vi "Begin.vi"(8 "error in (no error)":errorcluster, 11 "DriveMotors in":refnum<class "DriveMotors.lvclass">) -> (0 "error out":errorcluster, 3 "DriveMotors out":refnum<class "DriveMotors.lvclass">)   [LabVIEW 2013, in "DriveMotors.lvclass"]
uses:
  DriveMotors.lvclass
  DriveMotors.lvclass/DriveMotors.ctl
  System/System.lvclass
  <vilib>/Rock Robotics/WPI/Counter/WPI_CounterDigitalInputToDigitalSource.vi
  <vilib>/Rock Robotics/WPI/MotorControl/WPI_MotorControlOpenCANJaguar.vi
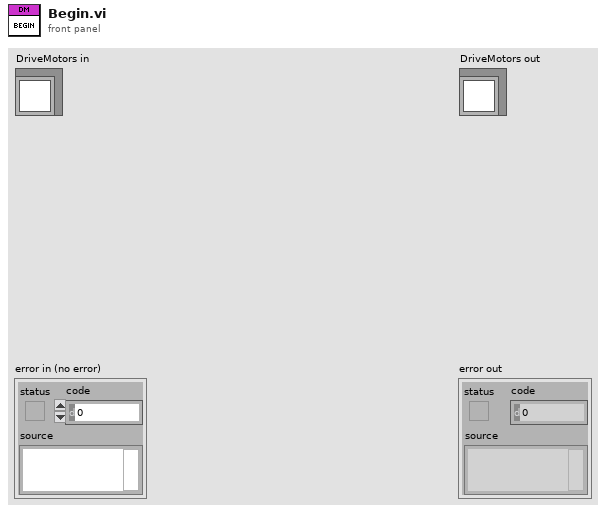
[diagram p1: front panel]
types:
  T1 = typedef "WPI_MotorControlDeviceRef.ctl" = cluster{"DeviceStatus":errorcluster, "Type":enum16{"PWM", "CAN"}, "PWM":cluster{"Digital Module":T2, "PWM Channel":T3, "DeadBand":T4}, "CAN":cluster{"Device Number":u8, "Control Mode":T5, "Semaphore":T6, "Max Vout":dbl}, "Invert":bool, "TransformRef":T7, "InvTransformRef":T7}
  T2 = typedef "FPGA_TypedefDigitalModule.ctl" = enum16{"Digital Module 1", "Digital Module 2"}
  T3 = typedef "FPGA_DIOPWMChannel.ctl" = enum8{"PWM 1", "PWM 2", "PWM 3", "PWM 4", "PWM 5", "PWM 6", "PWM 7", "PWM 8", "PWM 9", "PWM 10", "Invalid"}
  T4 = typedef "WPI_PWMDeadband.ctl" = cluster{"Name":string, "maxPositivePwm":i32, "minPositivePwm":i32, "centerPwm":i32, "maxNegativePwm":i32, "minNegativePwm":i32, "angularRange":u16}
  T5 = typedef "WPI_CANJaguar_ControlMode.ctl" = enum8{"Percent VBus", "Current", "Speed", "Position", "Voltage"}
  T6 = typedef "Semaphore RefNum" = refnum<k1>
  T7 = typedef "WPI_PWMTransform_ConPane.ctl" = refnum<vi>
  T8 = typedef "FPGA_DIOChannel.ctl" = enum8{"DIO 1", "DIO 2", "DIO 3", "DIO 4", "DIO 5", "DIO 6", "DIO 7", "DIO 8", "DIO 9", "DIO 10", "DIO 11", "DIO 12", "DIO 13", "DIO 14", "Invalid"}
  T9 = typedef "WPI_EncoderType.ctl" = enum16{"1x", "2x", "4x"}
  T10 = typedef "WPI_DigitalInputDevRef.ctl" = cluster{"DevStatus":errorcluster, "DIO Channel":T8, "Digital Module":T2}
  T11 = typedef "FPGA_CounterEncoderSourceConvertionLVSourceType.ctl" = cluster{"DevStatus":errorcluster, "AnalogTriggerMode?":bool, "DigitalMode":cluster{"Digital Module":T2, "DIO Channel":T12}, "AnalogTriggerMode":cluster{"AnalogTriggerIndex":T13, "OutputType":T14}}
  T12 = typedef "FPGA_DIODigitalSourceChannel.ctl" = enum8{"DIO 1", "DIO 2", "DIO 3", "DIO 4", "DIO 5", "DIO 6", "DIO 7", "DIO 8", "DIO 9", "DIO 10", "DIO 11", "DIO 12", "DIO 13", "DIO 14", "Disabled"}
  T13 = typedef "FPGA_AnalogTriggerIndex.ctl" = enum8{"Trig 0", "Trig 1", "Trig 2", "Trig 3", "Trig 4", "Trig 5", "Trig 6", "Trig 7", "Invalid"}
  T14 = typedef "FPGA_AnalogTriggerOutType.ctl" = enum16{"InWindow", "TriggerState", "Rising", "Falling"}
  T15 = typedef "WPI_EncoderDevRef.ctl" = cluster{"DevStatus":errorcluster, "EncoderIndex":T16, "CounterIndex":T17, "DistancePerCount":dbl, "Decoding Type":T9}
  T16 = typedef "FPGA_EncoderIdx.ctl" = enum8{"Enc 0", "Enc 1", "Enc 2", "Enc 3", "Invalid"}
  T17 = typedef "FPGA_CounterCtrSystemIndex.ctl" = enum8{"Ctr 0", "Ctr 1", "Ctr 2", "Ctr 3", "Ctr 4", "Ctr 5", "Ctr 6", "Ctr 7", "Invalid"}
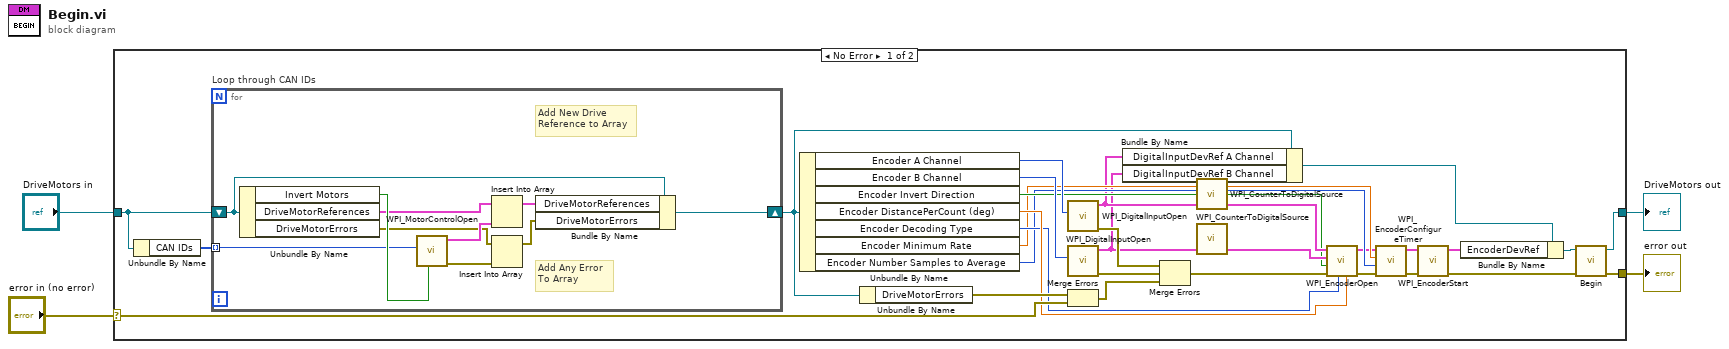
[diagram p0: block diagram]
diagram:
  n1 = case shown="No Error" "error in (no error)" {
    selector: "error in (no error)" -> [w30 w46]
    tunnel: [w29 w46] -> w3
    tunnel: [w32 w45] -> w1
    tunnel: "DriveMotors in" -> [w33 w45]
    frame No Error {
      n2 = Unbundle By Name(w33) -> ("CAN IDs"=w34:u8[])
      n3 = for "Loop through CAN IDs" {
        tunnel: w34 -> [w43] mode=indexing
        shift-right: [w41] -> w28
        shift-left: w33 -> [w42]
        # "Add Any Error\nTo Array"
        # "Add New Drive\nReference to Array"
        n4 = Unbundle By Name(w42) -> ("Invert Motors"=w44:bool, "DriveMotorReferences"=w40:T1[], "DriveMotorErrors"=w37:errorcluster[])
        n5 = call-poly <vilib>:"WPI_MotorControlOpen.vi"("Invert"=w44, "Device Number"=w43) -> ("error out"=w36:errorcluster, "MotorControlDeviceRef"=w39:T1)  [unwired: 8 in]
        n6 = Insert Into Array(array=w40, new element=w39) -> (w38:T1[])  [unwired: 1 in]
        n7 = Insert Into Array(array=w37, new element=w36) -> (w35:errorcluster[])  [unwired: 1 in]
        n8 = Bundle By Name(cluster=w42, "DriveMotorReferences"=w38, "DriveMotorErrors"=w35) -> (w41:refnum<class "DriveMotors.lvclass">)
      }
      n9 = Unbundle By Name(w28) -> ("Encoder A Channel"=w27:T8, "Encoder B Channel"=w26:T8, "Encoder Invert Direction"=w23:bool, "Encoder DistancePerCount (deg)"=w22:dbl, "Encoder Decoding Type"=w21:T9, "Encoder Minimum Rate"=w19:dbl, "Encoder Number Samples to Average"=w18:u8)
      n10 = Unbundle By Name(w28) -> ("DriveMotorErrors"=w31:errorcluster[])
      n11 = call <vilib>:"WPI_DigitalInputOpen.vi"("DIO Channel"=w27) -> ("error out"=w16:errorcluster, "DigitalInputDevRef"=w6:T10)  [unwired: 2 in, 7 out]
      n12 = call <vilib>:"WPI_DigitalInputOpen.vi"("DIO Channel"=w26) -> ("error out"=w15:errorcluster, "DigitalInputDevRef"=w5:T10)  [unwired: 2 in, 7 out]
      n13 = Merge Errors(w31, w30) -> (w14:errorcluster)
      n14 = Bundle By Name(cluster=w28, "DigitalInputDevRef A Channel"=w6, "DigitalInputDevRef B Channel"=w5) -> (w7:refnum<class "DriveMotors.lvclass">)
      n15 = Merge Errors(w16, w15, w14) -> (w13:errorcluster)
      n16 = call-poly <vilib>:"WPI_CounterToDigitalSource.vi"("DigitalInputDevRef"=w6) -> ("Digital Source"=w25:T11)  [unwired: 6 out]
      n17 = call-poly <vilib>:"WPI_CounterToDigitalSource.vi"("DigitalInputDevRef"=w5) -> ("Digital Source"=w24:T11)  [unwired: 6 out]
      n18 = call <vilib>:"WPI_EncoderOpen.vi"("DistancePerCount"=w22, "Decoding Type"=w21, "error in (no error)"=w13, "Invert Direction (False)"=w23, "BSource"=w24, "ASource"=w25) -> ("error out"=w12:errorcluster, "EncoderDevRef"=w17:T15)  [unwired: 2 in, 2 out]
      n19 = call <vilib>:"WPI_EncoderConfigureTimer.vi"("error in (no error)"=w12, "Number Samples to Average"=w18, "Minimum Rate"=w19, "EncoderDevRef"=w17) -> ("error out"=w11:errorcluster, "EncoderDevRef"=w9:T15)  [unwired: 6 out]
      n20 = call <vilib>:"WPI_EncoderStart.vi"("error in (no error)"=w11, "EncoderDevRef"=w9) -> ("error out"=w10:errorcluster, "EncoderDevRef"=w8:T15)  [unwired: 8 out]
      n21 = Bundle By Name(cluster=w7, "EncoderDevRef"=w8) -> (w20:refnum<class "DriveMotors.lvclass">)
      n22 = call-parent "Begin.vi"("error in (no error)"=w10, "System in"=w20) -> ("error out"=w29:errorcluster, "System out"=w32:refnum<class "DriveMotors.lvclass">)  [unwired: 8 in]
    }
    frame Error {
    }
  }
  "error out" <- w3
  "DriveMotors out" <- w1
